vi "Calling Python Objects from LabVIEW.vi"() -> ()   [LabVIEW 2024]
panel:
  in  "Input":dbl=1.0 format="%#_13g"
  in  "Increment Value":dbl=1.0 format="%#_13g"
  out "error out":errorcluster
  in  "error in":errorcluster
  out "Result":dbl
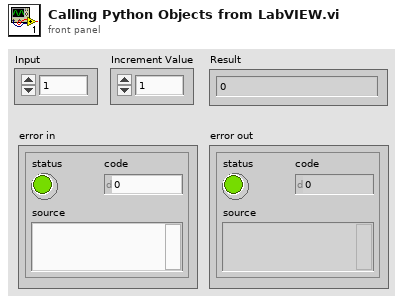
[diagram p1: front panel]
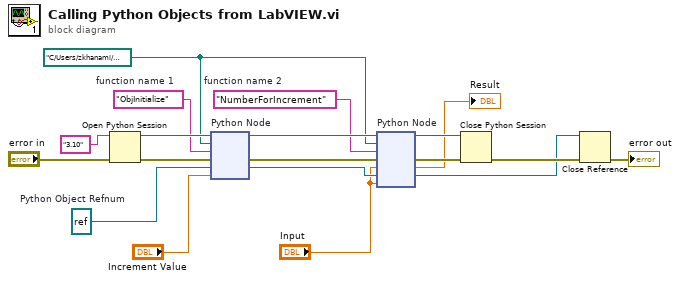
[diagram p0: block diagram]
diagram:
  w4 = path "C:/Users/zkhanami/Desktop/Solutions/Exercise 19-2 Calling Python Objects from LabVIEW/pyClass.py" ("module path")
  w6 = "NumberForIncrement"  # function name 2
  w7 = "ObjInitialize"  # function name 1
  w19 = refnum<k38> refnum  # Python Object Refnum
  n1 = Open Python Session(python version="3.10" ("Python version"), 3:"error in") -> (session out=w18:refnum<k35>, error out=w17:errorcluster)  [unwired: 1 in]
  n2 = node "Python Node"(w18, w4, w7, w17, w19, "Increment Value") -> (w15:refnum<k35>, w16:errorcluster, w11:refnum<k38>)  [unwired: 1 in, 2 out]
  n3 = node "Python Node"(w15, w4, w6, w16, "Input", w11, "Input") -> (w14:refnum<k35>, w13:errorcluster, →"Result":dbl, w10:refnum<k38>)  [unwired: 1 in, 2 out]
  n4 = Close Python Session(session in=w14, error in=w13) -> (11:w12:errorcluster)
  n5 = Close Reference(reference=w10, error in (no error)=w12) -> (error out=→"error out":errorcluster)
